vi "Module Not Running--error.vi"() -> (0 "error out":errorcluster)   [LabVIEW 2020, in "Module 1.lvlib"]
doc: "Outputs an error cluster containing a custom error code indicating the module is not running.\n_____\nBased on DQMH Project Template 6.0.0.91."
uses:
  Module 1.lvlib
  <vilib>/Utility/error.llb/Error Cluster From Error Code.vi
  <vilib>/ErrorRing/Error Ring.xnode
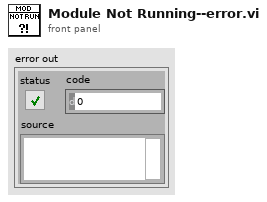
[diagram p1: front panel]
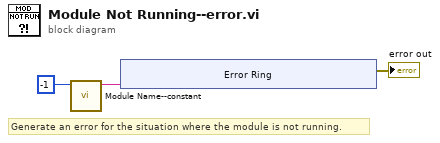
[diagram p0: block diagram]
diagram:
  # "Generate an error for the situation where the module is not running."
  n1 = call "Module Name--constant.vi"("Module ID"=-1) -> ("Module Name"=w1:string)  [unwired: 10 in]
  n2 = xnode "Error Ring"("parameter 0"=w1) -> ("error out"=→"error out":errorcluster)
